vi "Checa_Cupula.vi"(6 "ErroCupCustom":i16, 9 "Target":u16) -> (0 "sentido":bool, 1 "angCUP":string, 2 "moverCup":bool, 3 "angTarget":string)   [LabVIEW 2012]
uses:
  Global_Telescopio.vi
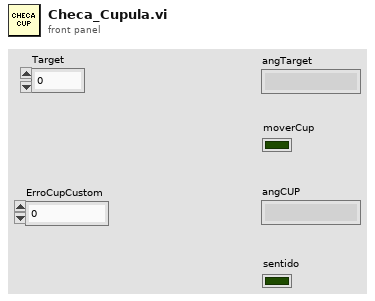
[diagram p1: front panel]
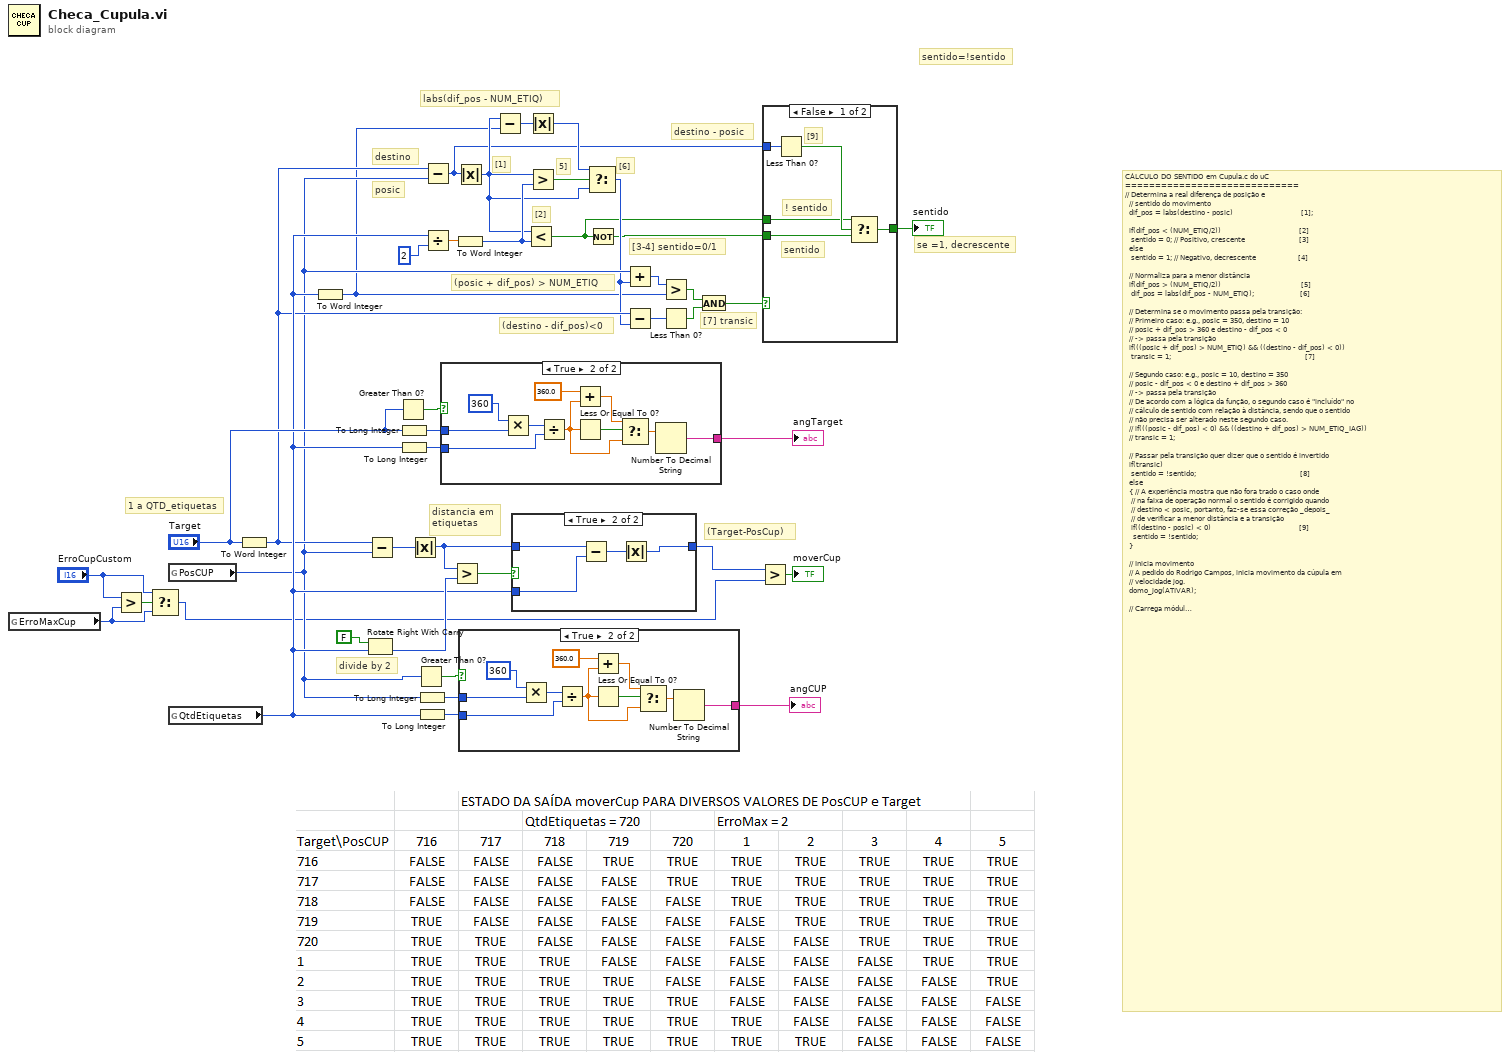
[diagram p0: block diagram]
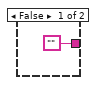
[diagram p3: hidden frame]
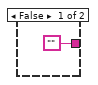
[diagram p4: hidden frame]
diagram:
  # "(Target-PosCup)"
  # "destino - posic"
  # "labs(dif_pos - NUM_ETIQ)"
  # "[6]"
  # "5]"
  # "sentido=!sentido"
  # "[2]"
  # "[1]"
  # "posic"
  # "destino"
  # "[3-4] sentido=0/1"
  # "[7] transic"
  # "(posic + dif_pos) > NUM_ETIQ"
  # "(destino - dif_pos)<0"
  # "se =1, decrescente"
  # "CÁLCULO DO SENTIDO em Cupula.c do uC\n=============================\t\t\n// Determina a real diferença de posição e\n\t\t// sentido do movimento\n\t\tdif_pos = labs(destino - posic)                                  [1];\n\n\t\tif(dif_pos < (NUM_ETIQ/2))                                       [2]\n\t\t\tsentido = 0;\t// Positivo, crescente                           [3]\n\t\telse\n\t\t\tsentido = 1;\t// Negativo, decrescente                     [4]\n\t\n\t\t// Normaliza para a menor distância\n\t\tif(dif_pos > (NUM_ETIQ/2))                                        [5]\n\t\t\tdif_pos = labs(dif_pos - NUM_ETIQ);                       [6]\n\n\t\t// Determina se o movimento passa pela transição:\n\t\t// Primeiro caso: e.g., posic = 350, destino = 10\n\t\t// posic + dif_pos > 360 e destino - dif_pos < 0 \n\t\t// -> passa pela transição\n\t\tif(((posic + dif_pos) > NUM_ETIQ) && ((destino - dif_pos) < 0))\n\t\t\ttransic = 1;                                                                   [7]\n\n\t\t// Segundo caso: e.g., posic = 10, destino = 350\n\t\t// posic - dif_pos < 0 e destino + dif_pos > 360\n\t\t// -> passa pela transição\n\t\t// De acordo com a lógica da função, o segundo caso é \"incluído\" no\n\t\t// cálculo de sentido com relação à distância, sendo que o sentido\n\t\t// não precisa ser alterado neste segundo caso.\n\t\t// if(((posic - dif_pos) < 0) && ((destino + dif_pos) > NUM_ETIQ_IAG))\n\t\t//\ttransic = 1;\n\n\t\t// Passar pela transição quer dizer que o sentido é invertido\n\t\tif(transic)\n\t\t\tsentido = !sentido;                                                    [8]\n\t\telse\n\t\t{\t// A experiência mostra que não fora trado o caso onde\n\t\t\t// na faixa de operação normal o sentido é corrigido quando\n\t\t\t// destino < posic, portanto, faz-se essa correção _depois_\n\t\t\t// de verificar a menor distância e a transição\n\t\t\tif((destino - posic) < 0)                                            [9]\n\t\t\t\tsentido = !sentido;\n\t\t}\n\n\t\t// Inicia movimento\n\t\t// A pedido do Rodrigo Campos, inicia movimento da cúpula em\n\t\t// velocidade jog.\n\t\tdomo_jog(ATIVAR);\n\n\t\t// Carrega módulo TIMEOUT1 com 4s.\n\t\tset_timeout(1,200,1);\n\n\t\tif(!sentido)\n\t\t\tdomo_pos(ATIVAR);\n\t\telse\n\t\t\tdomo_neg(ATIVAR);"
  # "divide by 2"
  # "1 a QTD_etiquetas"
  # "distancia em\netiquetas"
  n1 = global read "Global_Telescopio.vi" "ErroMaxCup"() -> (w2:i16)
  n2 = Greater?(x="ErroCupCustom", y=w2) -> (0:w4:bool)
  n3 = Select(t="ErroCupCustom", s=w4, f=w2) -> (s? t:f=w1:i16)
  n4 = global read "Global_Telescopio.vi" "PosCUP"() -> (w15:i16)
  n5 = global read "Global_Telescopio.vi" "QtdEtiquetas"() -> (w25:i16)
  n6 = To Word Integer(number="Target") -> (16bit integer=w17:i16)
  n7 = To Word Integer(number=w25) -> (16bit integer=w12:i16)
  n8 = Rotate Right With Carry(2:w25, 3:FALSE ("carry")) -> (0:w34:i16)  [unwired: 1 out]
  n9 = Subtract(x=w17, y=w15) -> (x-y=w37:i16)
  n10 = Greater Than 0?(x="Target") -> (x > 0?=w28:bool)
  n11 = To Long Integer(number="Target") -> (32bit integer=w30:i32)
  n12 = To Long Integer(number=w25) -> (32bit integer=w29:i32)
  n13 = Absolute Value(x=w37) -> (abs(x)=w40:i16)
  n14 = Greater Than 0?(x=w15) -> (x > 0?=w33:bool)
  n15 = To Long Integer(number=w15) -> (32bit integer=w31:i32)
  n16 = To Long Integer(number=w25) -> (32bit integer=w32:i32)
  n17 = Subtract(x=w17, y=w15) -> (x-y=w6:i16)
  n18 = Divide(x=w25, y=i16 2) -> (x/y=w23:dbl)
  n19 = case shown="True" w28 {
    tunnel: ["" w51] -> w27
    tunnel: w29 -> [_ w44]
    tunnel: w30 -> [_ w43]
    frame False {
    }
    frame True {
      n20 = Multiply(x=360, y=w43) -> (x*y=w50:i32)
      n21 = Divide(x=w50, y=w44) -> (x/y=w47:dbl)
      n22 = Add(x=360.0, y=w47) -> (x+y=w45:dbl)
      n23 = Less Or Equal To 0?(x=w47) -> (x <= 0?=w49:bool)
      n24 = Select(t=w45, s=w49, f=w47) -> (s? t:f=w48:dbl)
      n25 = Number To Decimal String(number=w48) -> (decimal integer string=w51:string)  [unwired: 1 in]
    }
  }
  "angTarget" <- w27
  n26 = Greater?(x=w40, y=w34) -> (0:w41:bool)
  n27 = To Word Integer(number=w23) -> (16bit integer=w22:i16)
  n28 = Absolute Value(x=w6) -> (abs(x)=w18:i16)
  n29 = case shown="True" w33 {
    tunnel: ["" w62] -> w36
    tunnel: w32 -> [_ w55]
    tunnel: w31 -> [_ w54]
    frame False {
    }
    frame True {
      n30 = Multiply(x=360, y=w54) -> (x*y=w61:i32)
      n31 = Divide(x=w61, y=w55) -> (x/y=w58:dbl)
      n32 = Add(x=360.0, y=w58) -> (x+y=w56:dbl)
      n33 = Less Or Equal To 0?(x=w58) -> (x <= 0?=w60:bool)
      n34 = Select(t=w56, s=w60, f=w58) -> (s? t:f=w59:dbl)
      n35 = Number To Decimal String(number=w59) -> (decimal integer string=w62:string)  [unwired: 1 in]
    }
  }
  "angCUP" <- w36
  n36 = Subtract(x=w18, y=w12) -> (x-y=w19:i16)
  n37 = case shown="True" w41 {
    tunnel: w40 -> [w64 w68]
    tunnel: [w64 w66] -> w39
    tunnel: w25 -> [_ w65]
    frame False {
    }
    frame True {
      n38 = Subtract(x=w68, y=w65) -> (x-y=w67:i16)
      n39 = Absolute Value(x=w67) -> (abs(x)=w66:i16)
    }
  }
  n40 = Less?(x=w18, y=w22) -> (x < y?=w8:bool)
  n41 = Absolute Value(x=w19) -> (abs(x)=w20:i16)
  n42 = Greater?(x=w18, y=w22) -> (0:w21:bool)
  n43 = Select(t=w20, s=w21, f=w18) -> (s? t:f=w14:i16)
  n44 = Not(x=w8) -> (.not. x?=w9:bool)
  n45 = Add(x=w15, y=w14) -> (x+y=w13:i16)
  n46 = Subtract(x=w17, y=w14) -> (x-y=w16:i16)
  n47 = Greater?(x=w13, y=w12) -> (0:w10:bool)
  n48 = Less Than 0?(x=w16) -> (x < 0?=w11:bool)
  n49 = And(x=w10, y=w11) -> (x .and. y?=w7:bool)
  n50 = Greater?(x=w39, y=w1) -> (0:→"moverCup":bool)
  n51 = case shown="False" w7 {
    tunnel: w9 -> [w70 _]
    tunnel: w8 -> [w71 w74]
    tunnel: w6 -> [w73 _]
    tunnel: [w69 w74] -> w5
    frame False {
      # "sentido"
      # "! sentido"
      # "[9]"
      n52 = Less Than 0?(x=w73) -> (x < 0?=w72:bool)
      n53 = Select(t=w71, s=w72, f=w70) -> (s? t:f=w69:bool)
    }
    frame True {
      # "[8]"
    }
  }
  "sentido" <- w5
